vi "start.vi"(8 "error in (no error)":errorcluster, 11 "Model in":refnum<class "Model.lvclass">) -> (0 "error out":errorcluster, 3 "Model out":refnum<class "Model.lvclass">)   [LabVIEW 2013, in "Model.lvclass"]
uses:
  Model.lvclass
  Model.lvclass/Model.ctl
  <userlib>/Common/ILC/ILC/ILC.lvclass
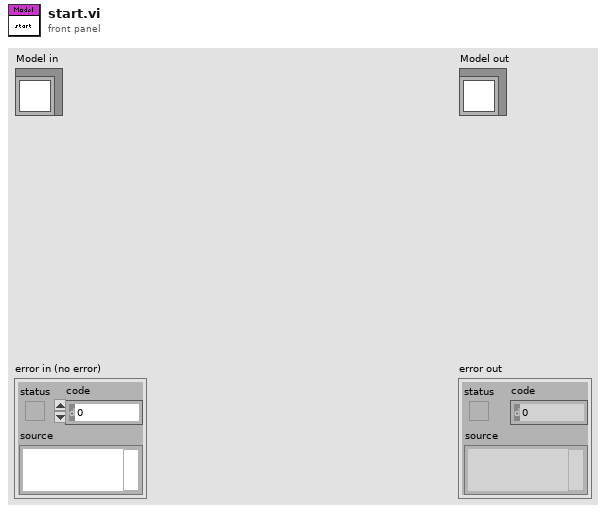
[diagram p1: front panel]
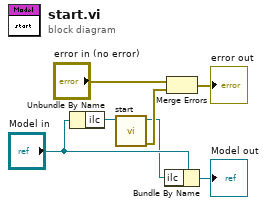
[diagram p0: block diagram]
diagram:
  n1 = Unbundle By Name("Model in") -> ("ilc"=w5:refnum<class "ILC.lvclass">)
  n2 = call <userlib>:"start.vi"("ILC in"=w5) -> ("error out"=w4:errorcluster, "ILC out"=w1:refnum<class "ILC.lvclass">)  [unwired: 9 in]
  n3 = Bundle By Name(cluster="Model in", "ilc"=w1) -> (→"Model out":refnum<class "Model.lvclass">)
  n4 = Merge Errors("error in (no error)", w4) -> (→"error out":errorcluster)
